vi "StartChannel.vi"(8 "error in (no error)":errorcluster, 10 "Channel":u8, 11 "ID In":i32) -> (0 "error out":errorcluster, 3 "ID Out":i32)   [LabVIEW 2022 SP3, in "EClib functions.lvlib"]
doc: "This VI start loaded ecc protocols on the selected channel."
uses:
  EClib functions.lvlib
panel:
  out "arg1":i32
  out "arg2":u8
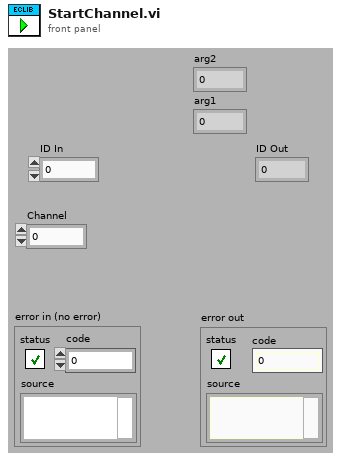
[diagram p1: front panel]
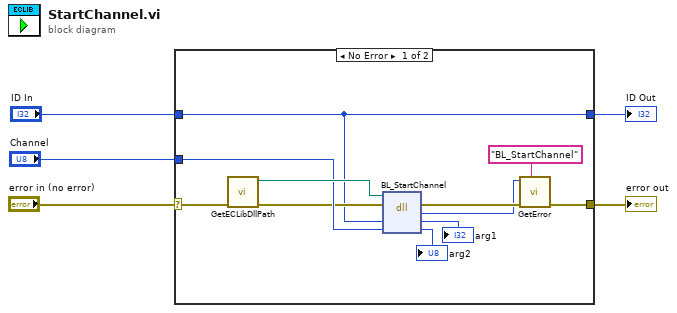
[diagram p0: block diagram]
diagram:
  n1 = case shown="No Error" "error in (no error)" {
    selector: "error in (no error)" -> [w14 w18]
    tunnel: [w8 w18] -> w5
    tunnel: "ID In" -> [w9 w17]
    tunnel: "Channel" -> [w15 _]
    tunnel: [w9 w17] -> w1
    frame No Error {
      n2 = call "GetECLibDllPath.vi"("error in (no error)"=w14) -> ("error out"=w13:errorcluster, "ECLibDLLPath"=w16:path)  [unwired: 9 in]
      n3 = dll-call lib="?" fn="BL_StartChannel"(path in=w16, error in=w13, "arg1"=w9, "arg2"=w15) -> (error out=w12:errorcluster, "return type"=w10:i32, "arg1"=→"arg1":i32, "arg2"=→"arg2":u8)  [unwired: 1 in, 1 out]
      n4 = call "GetError.vi"("DLLFunction"="BL_StartChannel", "error in"=w12, "code"=w10) -> ("error out"=w8:errorcluster)  [unwired: 8 in]
    }
    frame Error {
    }
  }
  "error out" <- w5
  "ID Out" <- w1
